vi "Send Trigger Settings.vi"(8 "error in (no error)":errorcluster, 11 "5105 in":refnum<class "5105.lvclass">) -> (0 "error out":errorcluster, 3 "5105 out":refnum<class "5105.lvclass">)   [LabVIEW 2019, in "5105.lvlib" / "5105.lvclass"]
uses:
  5105.lvclass
  C:/Users/Public/Documents/Development/builds/Instruments/Oscilloscope.lvlibp/Oscilloscope.lvclass
  <instrlib>/niScope/Controls/niScope trigger source.ctl
  Accessors/Read Local Resource.vi
  builds/Instruments/Oscilloscope.lvlibp/Accessors/Read Trigger Settings.vi
  <instrlib>/niScope/Configure/Trigger/niScope Configure Trigger Immediate.vi
  <instrlib>/niScope/Configure/Trigger/niScope Configure Trigger Edge.vi
  <instrlib>/niScope/Configure/Trigger/niScope Configure Trigger Digital.vi
  Accessors/Write Local Resource.vi
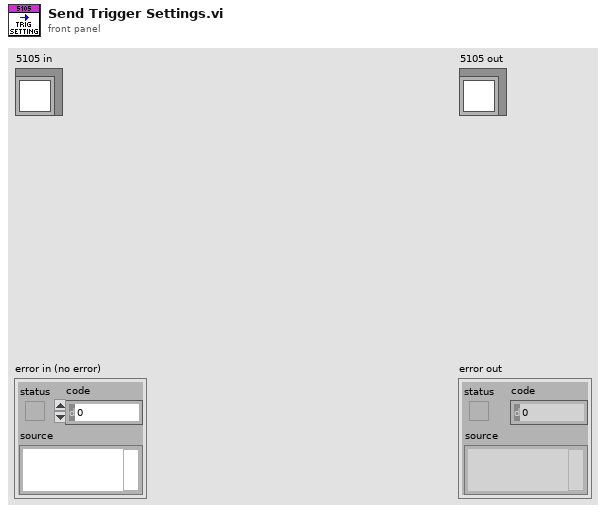
[diagram p1: front panel]
types:
  T1 = typedef "Oscilloscope.lvlibp/Oscilloscope.lvclass/Trigger Settings.ctl" = cluster{"Edge:":T2, "Level":dbl, "Source":T3, "trigger coupling":T4, "Holdoff":dbl, "Delay":dbl, "Trigger Modifier":T5, "Trigger Type":T6}
  T2 = typedef "Oscilloscope.lvlibp/Oscilloscope.lvclass/Edge Select.ctl" = u16
  T3 = typedef "Oscilloscope.lvlibp/Oscilloscope.lvclass/Channel List.ctl" = u16
  T4 = typedef "Oscilloscope.lvlibp/Oscilloscope.lvclass/Trigger Coupling.ctl" = u16
  T5 = typedef "Oscilloscope.lvlibp/Oscilloscope.lvclass/Trigger Modifier.ctl" = enum16{"Invalid_Setting", "None", "Auto Trigger"}
  T6 = typedef "Oscilloscope.lvlibp/Oscilloscope.lvclass/Trigger Type.ctl" = enum16{"Immediate", "Analog Edge", "Digital", "Window", "Hysteresis"}
  T7 = typedef "niScope trigger source.ctl" = string
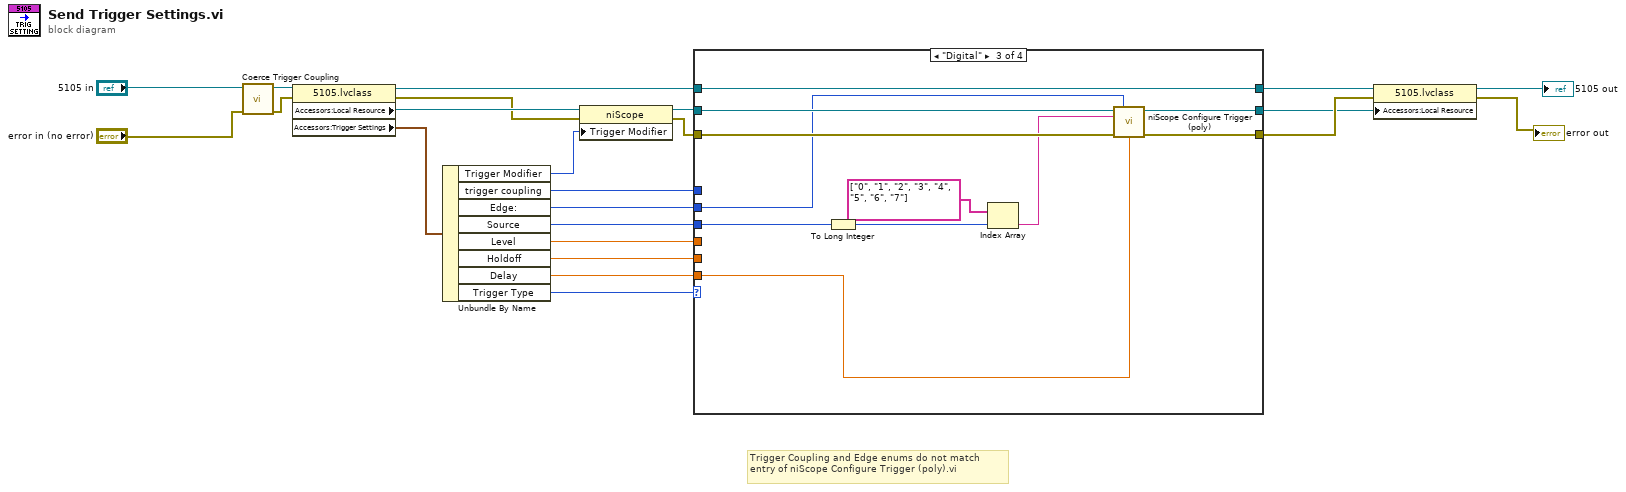
[diagram p0: block diagram]
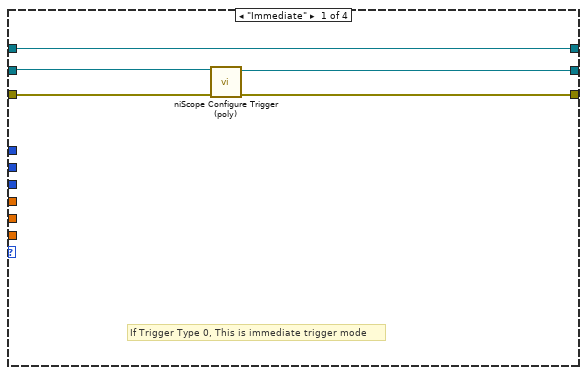
[diagram p2: hidden frame]
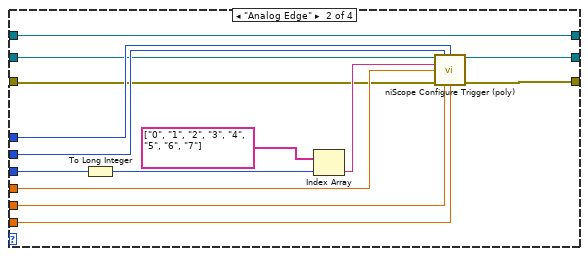
[diagram p3: hidden frame]
diagram:
  # "Trigger Coupling and Edge enums do not match entry of niScope Configure Trigger (poly).vi"
  n1 = call "Coerce Trigger Coupling.vi"("error in (no error)"="error in (no error)", "5105 in"="5105 in") -> ("error out"=w18:errorcluster, "5105 out"=w20:refnum<class "5105.lvclass">)  [unwired: 8 in]
  n2 = property class="5105.lvclass"(reference=w20, error in=w18) -> (reference out=w16:refnum<class "5105.lvclass">, error out=w14:errorcluster, "Accessors:Local Resource"=w15:refnum<k15>, "Accessors:Trigger Settings"=w17:T1)
  n3 = Unbundle By Name(w17) -> ("Trigger Modifier"=w1:T5, "trigger coupling"=w7:T4, "Edge:"=w6:T2, "Source"=w8:T3, "Level"=w5:dbl, "Holdoff"=w4:dbl, "Delay"=w9:dbl, "Trigger Type"=w10:T6)
  n4 = property class="niScope"(reference=w15, error in=w14, "Trigger Modifier"=w1) -> (reference out=w3:refnum<k15>, error out=w2:errorcluster)
  n5 = case shown="\"Digital\"" w10 {
    tunnel: w2 -> [w28 w29 w53 w55]
    tunnel: [w27 w42 w52 w55] -> w13
    tunnel: [w26 w41 w51 w54] -> w11
    tunnel: w3 -> [w24 w30 w47 w54]
    tunnel: w16 -> [w25 w37 w46 w56]
    tunnel: [w25 w37 w46 w56] -> w12
    tunnel: w9 -> [_ w31 w43 _]
    tunnel: w8 -> [_ w34 w44 _]
    tunnel: w7 -> [_ w36 _ _]
    tunnel: w6 -> [_ w35 w45 _]
    tunnel: w5 -> [_ w33 _ _]
    tunnel: w4 -> [_ w32 _ _]
    frame "Immediate" {
      # "If Trigger Type 0, This is immediate trigger mode"
      n6 = call-poly <instrlib>:"niScope Configure Trigger (poly).vi"("instrument handle"=w24, "error in"=w28) -> ("instrument handle out"=w26:refnum<k15>, "error out"=w27:errorcluster)  [unwired: 12 in]
    }
    frame "Analog Edge" {
      n7 = To Long Integer(number=w34) -> (32bit integer=w39:i32)
      n8 = Index Array(array=T7[] ["0", "1", "2", "3", "4", "5", "6", "7"], index=w39) -> (element=w38:T7)
      n9 = call-poly <instrlib>:"niScope Configure Trigger (poly).vi"("instrument handle"=w30, "trigger slope"=w35, "trigger coupling"=w36, "trigger source"=w38, "trigger level"=w33, "error in"=w29, "trigger holdoff"=w32, "trigger delay"=w31) -> ("instrument handle out"=w41:refnum<k15>, "error out"=w42:errorcluster)  [unwired: 6 in]
    }
    frame "Digital" {
      n10 = To Long Integer(number=w44) -> (32bit integer=w49:i32)
      n11 = Index Array(array=T7[] ["0", "1", "2", "3", "4", "5", "6", "7"], index=w49) -> (element=w48:T7)
      n12 = call-poly <instrlib>:"niScope Configure Trigger (poly).vi"("instrument handle"=w47, "trigger slope"=w45, "trigger source"=w48, "error in"=w53, "trigger delay"=w43) -> ("instrument handle out"=w51:refnum<k15>, "error out"=w52:errorcluster)  [unwired: 9 in]
    }
    frame Default {
    }
  }
  n13 = property class="5105.lvclass"(reference=w12, error in=w13, "Accessors:Local Resource"=w11) -> (reference out=→"5105 out":refnum<class "5105.lvclass">, error out=→"error out":errorcluster)
